vi "Disarm Command.vi"(8 "error in (no error)":errorcluster, 10 "Request type":T1, 11 "Pulse Controller in":refnum<class "Pulse Controller.lvclass">) -> (0 "error out":errorcluster, 3 "Pulse Controller out":refnum<class "Pulse Controller.lvclass">)   [LabVIEW 2021, in "Pulse Controller.lvclass"]
uses:
  Pulse Controller.lvclass
  C:/GitHub/LabActor/Worker/Worker Actor/Worker Actor.lvclass
  C:/GitHub/LabActor/Template Module/Template Module.lvclass
  C:/Program Files/National Instruments/LabVIEW 2021/vi.lib/ActorFramework/Actor/Actor.lvclass
  C:/GitHub/LabActor/Controllers/Process Controller/Process Controller.lvclass
  Process Controller/Request type.ctl
  Worker/Worker Actor/Worker Actor.lvclass/Worker Actor.ctl
  NHMFL_Core/Libraries/Instruments/Instrument Driver/Worker State.ctl
  NHMFL_Core/Libraries/Instruments/Results/File Path Result/File Path Result.lvclass
  C:/GitHub/NHMFL_Core/Libraries/Instruments/Results/Acquired Result/Acquired Result.lvclass
  Template Module/Template Module.lvclass/Template Module.ctl
  NHMFL_Core/Libraries/Instruments/Results/Acquired Result/Acquired Result.lvclass/Acquired Result.ctl
  Pulse Controller.lvclass/Pulse Controller.ctl
  <vilib>/ActorFramework/Actor/Actor.lvclass/Actor.ctl
  Interfaces/Application Messages/New Pulse Acquired Msg/New Pulse Acquired Msg.lvclass/New Pulse Acquired Msg.ctl
  <vilib>/ActorFramework/Message Enqueuer/Message Enqueuer.lvclass/Message Enqueuer.ctl
  Process Controller/Process Controller.lvclass/Process Controller.ctl
  Pulse Recorders/Interfaces/Pulse Recorder Messages/Disarm Msg/Disarm Msg.lvclass/Disarm Msg.ctl
  Template Module/Read Logger.vi
  Template Module/Read Name.vi
  NHMFL_Core/Libraries/Instruments/Results/Acquired Result/Write Sender.vi
  Template Module/Write Logger.vi
  Process Controller/Read Active measurements enqueuers.vi
  Template Module/Write State.vi
  Template Module/Read tdms stream.vi
  Template Module/Read State.vi
  <vilib>/ActorFramework/Message Enqueuer/Enqueue.vi
  Interfaces/Application Messages/New Pulse Acquired Msg/New Pulse Acquired Msg.lvclass
  C:/Program Files/National Instruments/LabVIEW 2021/vi.lib/ActorFramework/Message/Message.lvclass
  Pulse Recorders/Interfaces/Pulse Recorder Messages/Disarm Msg/Disarm Msg.lvclass
  Read Pulse Controller Configuration.vi
  <vilib>/ActorFramework/Message Priority Queue/Priority Enqueue.vi
  Loggers/Logger/Logger.lvclass
  <vilib>/ActorFramework/Message Enqueuer/Message Enqueuer.lvclass
  <vilib>/ActorFramework/Actor/Actor.lvclass
  Template Module Messages/Result Reply Msg/Result Reply Msg.lvclass
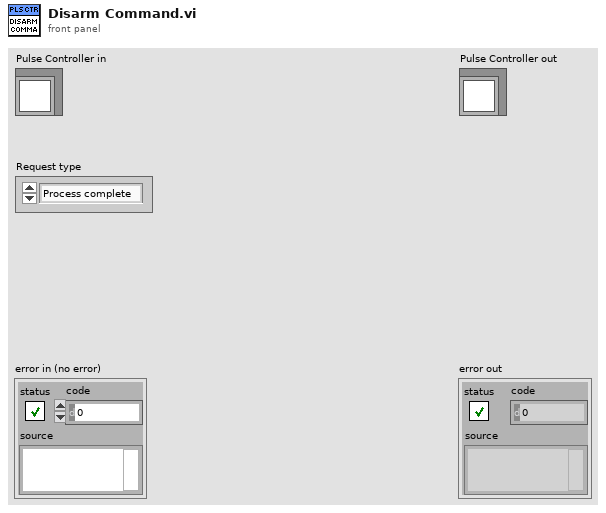
[diagram p1: front panel]
types:
  T1 = typedef "Request type.ctl" = enum16{"Process complete", "User command", "Auto-restart", "Error"}
  T2 = typedef "Worker State.ctl" = enum16{"Idle", "Starting", "Working", "Stopping"}
  T3 = typedef "Pulse Controller Configuration.ctl" = cluster{"Pre-trigger duration":dbl, "Post-trigger duration":dbl, "Open plot after pulse":bool, "Auto-rearm":bool, "Back-up raw data":bool}
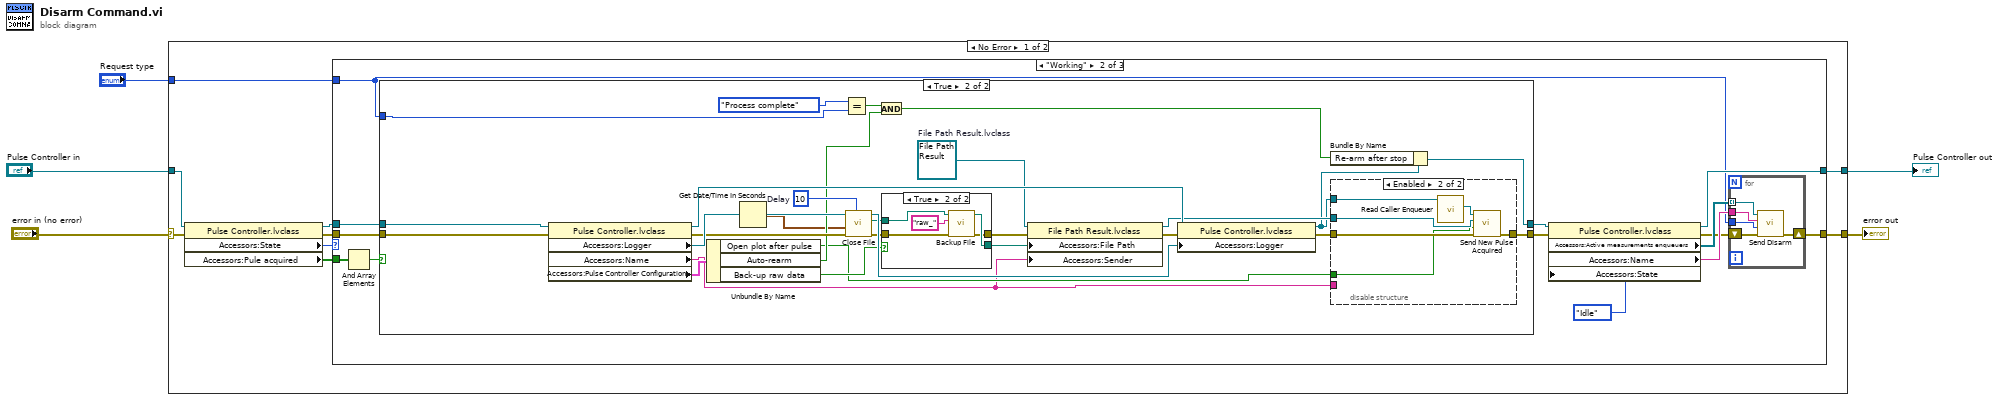
[diagram p0: block diagram]
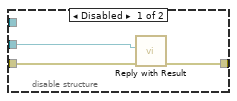
[diagram p4: hidden frame]
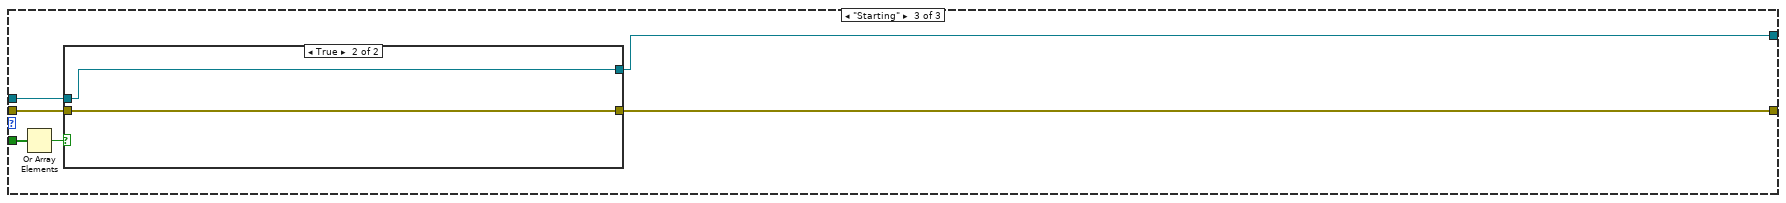
[diagram p6: hidden frame]
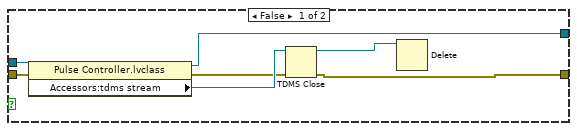
[diagram p7: hidden frame]
diagram:
  n1 = case shown="No Error" "error in (no error)" {
    selector: "error in (no error)" -> [w7 w98]
    tunnel: [w8 w98] -> w4
    tunnel: [w10 w97] -> w2
    tunnel: "Pulse Controller in" -> [w9 w97]
    tunnel: "Request type" -> [w11 _]
    frame No Error {
      n2 = property class="Pulse Controller.lvclass"(reference=w9, error in=w7) -> (reference out=w13:refnum<class "Pulse Controller.lvclass">, error out=w12:errorcluster, "Accessors:State"=w14:T2, "Accessors:Pule acquired"=w6:bool[])
      n3 = case shown="\"Working\"" w14 {
        tunnel: w13 -> [w15 w28 w84]
        tunnel: w12 -> [w16 w27 w83]
        tunnel: [w15 w22 w87] -> w10
        tunnel: [w16 w26 w86] -> w8
        tunnel: w11 -> [_ w18 _]
        tunnel: w6 -> [_ w21 w82]
        frame "Idle", Default {
        }
        frame "Working" {
          n4 = And Array Elements(Boolean array=w21) -> (logical AND=w29:bool)
          n5 = case shown="True" w29 {
            tunnel: [w36 w48] -> w25
            tunnel: [w35 w47] -> w20
            tunnel: w28 -> [w36 w56]
            tunnel: w27 -> [w35 w55]
            tunnel: w18 -> [_ w51]
            frame False {
            }
            frame True {
              w53 = u32 10  # Delay
              w60 = refnum<class "File Path Result.lvclass"> refnum  # File Path Result.lvclass
              n6 = property class="Pulse Controller.lvclass"(reference=w56, error in=w55) -> (reference out=w61:refnum<class "Pulse Controller.lvclass">, error out=w63:errorcluster, "Accessors:Logger"=w64:refnum<class "Logger.lvclass">, "Accessors:Name"=w38:string, "Accessors:Pulse Controller Configuration"=w62:T3)
              n7 = Unbundle By Name(w62) -> ("Open plot after pulse"=w39:bool, "Auto-rearm"=w49:bool, "Back-up raw data"=w41:bool)
              n8 = Get Date/Time In Seconds() -> (seconds since 1Jan1904=w37:timestamp)
              n9 = Equal?(x=Request_type."Process complete" ("Request type"), y=w51) -> (x = y?=w50:bool)
              n10 = call-dynamic "Close File.vi"("Delay"=w53, "error in (no error)"=w63, "Time Stamp"=w37, "Logger in"=w64) -> ("error out"=w43:errorcluster, "File Path"=w45:path, "Logger out"=w54:refnum<class "Logger.lvclass">)  [unwired: 4 in, 1 out]
              n11 = And(x=w50, y=w49) -> (x .and. y?=w46:bool)
              n12 = case shown="True" w41 {
                tunnel: w45 -> [w75 w80]
                tunnel: [w75 w79] -> w44
                tunnel: w43 -> [w76 w78]
                tunnel: [w76 w77] -> w42
                frame False {
                }
                frame True {
                  n13 = call "Backup File.vi"("Error In"=w78, "Prefix"="raw_", "File"=w80) -> ("Error Out"=w77:errorcluster, "Duplicate file"=w79:path)  [unwired: 6 in, 1 out]
                }
              }
              n14 = property class="File Path Result.lvclass"(reference=w60, error in=w42, "Accessors:File Path"=w44, "Accessors:Sender"=w38) -> (reference out=w57:refnum<class "File Path Result.lvclass">, error out=w59:errorcluster)
              n15 = property class="Pulse Controller.lvclass"(reference=w61, error in=w59, "Accessors:Logger"=w54) -> (reference out=w40:refnum<class "Pulse Controller.lvclass">, error out=w58:errorcluster)
              n16 = Bundle By Name(cluster=w40, "Re-arm after stop"=w46) -> (w48:refnum<class "Pulse Controller.lvclass">)
              n17 = disable-structure shown="Enabled" {
                disable-tunnel: w58 -> [w68 w70]
                disable-tunnel: w57 -> [w67 w72]
                disable-tunnel: [w66 w71] -> w47
                disable-tunnel: w38 -> [_ _]
                disable-tunnel: w40 -> [_ w74]
                disable-tunnel: w39 -> [_ w69]
                frame Disabled {
                  n18 = call-dynamic "Reply with Result.vi"("error in (no error)"=w68, "Result"=w67) -> ("error out"=w66:errorcluster, "Result Reply Msg in"=w65:refnum<class "Result Reply Msg.lvclass">)  [unwired: 7 in, 1 out]
                }
                frame Enabled {
                  n19 = call <vilib>:"Read Caller Enqueuer.vi"("Actor"=w74) -> ("Caller Enqueuer"=w73:refnum<class "Message Enqueuer.lvclass">)  [unwired: 10 in]
                  n20 = call "Send New Pulse Acquired.vi"("error in (no error)"=w70, "Open plot"=w69, "Result"=w72, "Message Enqueuer"=w73) -> ("error out"=w71:errorcluster)  [unwired: 6 in, 1 out]
                }
              }
            }
          }
          n21 = property class="Pulse Controller.lvclass"(reference=w25, error in=w20, "Accessors:State"=Worker_State."Idle" ("State")) -> (reference out=w22:refnum<class "Pulse Controller.lvclass">, error out=w19:errorcluster, "Accessors:Active measurements enqueuers"=w23:refnum<class "Message Enqueuer.lvclass">[], "Accessors:Name"=w24:string)
          n22 = for {
            tunnel: w23 -> [w34] mode=indexing
            shift-right: [w32] -> w26
            shift-left: w19 -> [w33]
            tunnel: w24 -> [w31]
            tunnel: w18 -> [w30]
            n23 = call "Send Disarm.vi"("error in (no error)"=w33, "Request type"=w30, "Requester"=w31, "Message Enqueuer"=w34) -> ("error out"=w32:errorcluster)  [unwired: 6 in, 1 out]
          }
        }
        frame "Starting" {
          n24 = Or Array Elements(Boolean array=w82) -> (logical OR=w85:bool)
          n25 = case shown="True" w85 {
            tunnel: [w92 w96] -> w87
            tunnel: [w91 w95] -> w86
            tunnel: w84 -> [w90 w96]
            tunnel: w83 -> [w89 w95]
            frame False {
              n26 = property class="Pulse Controller.lvclass"(reference=w90, error in=w89) -> (reference out=w92:refnum<class "Pulse Controller.lvclass">, error out=w93:errorcluster, "Accessors:tdms stream"=w94:refnum<k34>)
              n27 = TDMS Close(8:w93, 11:w94) -> (0:w91:errorcluster, 3:w88:path)
              n28 = Delete(path (use dialog)=w88) -> ()  [unwired: 4 in, 3 out]
            }
            frame True {
            }
          }
        }
      }
    }
    frame Error {
    }
  }
  "error out" <- w4
  "Pulse Controller out" <- w2
